vi "LEP_RV_StartInit.vi"(8 "error in (no error)":errorcluster, 9 "Application Name":string, 10 "Target Name":string, 11 "buildSpec ID":string) -> (0 "error out":errorcluster)   [LabVIEW 2011]
doc: "Download and execute built VxWorks downloadable module and attach the LabVIEW Embedded debuger."
uses:
  <vilib>/LabVIEW Targets/Embedded/ASWServer/MPU_ASWServer_GeneralIcons.ctl
  <vilib>/LabVIEW Targets/Embedded/ASWServer/MPU_ASWServer_GeneralCtrls.ctl
  <vilib>/LabVIEW Targets/Embedded/ASWServer/MPU_ASWServer_General_SetProgressBarTitle.vi
  <vilib>/LabVIEW Targets/Embedded/ASWServer/MPU_ASWServer_General_SetProgressBarValue.vi
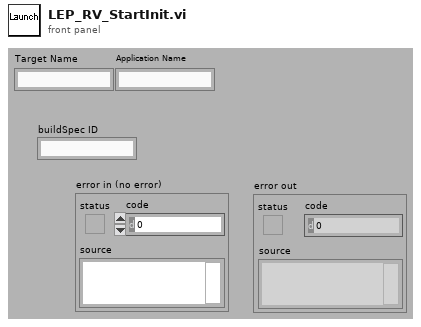
[diagram p1: front panel]
types:
  T1 = typedef "MPU_ASWServer_GeneralIcons.ctl" = enum16{"Complete", "Disconnected", "Error", "Initializing", "Ready", "Running", "Stopped", "Unknown", "No Change"}
  T2 = typedef "MPU_ASWServer_GeneralCtrls.ctl" = enum16{"Build Status", "Download Status", "Target Name", "Target Type", "Application Name"}
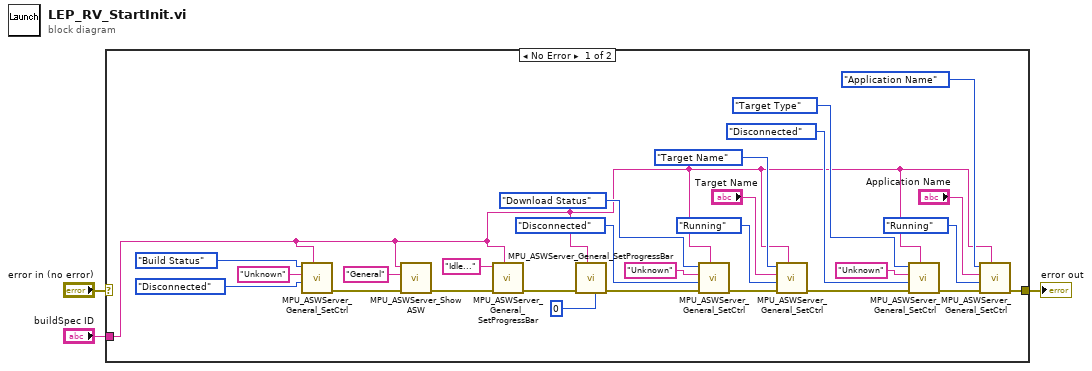
[diagram p0: block diagram]
diagram:
  n1 = case shown="No Error" "error in (no error)" {
    selector: "error in (no error)" -> [_ w31]
    tunnel: [w6 w31] -> w3
    tunnel: "buildSpec ID" -> [w8 _]
    frame No Error {
      n2 = call <vilib>:"MPU_ASWServer_General_SetCtrl.vi"("buildSpec ID"=w8, "icon"=MPU_ASWServer_GeneralIcons."Disconnected", "value"="Unknown", "control"=MPU_ASWServer_GeneralCtrls."Build Status") -> ("error out"=w5:errorcluster)  [unwired: 5 in, 2 out]
      n3 = call <vilib>:"MPU_ASWServer_Show ASW.vi"("error in (no error)"=w5, "tab name"="General", "buildSpec ID"=w8) -> ("error out"=w4:errorcluster)  [unwired: 7 in, 1 out]
      n4 = call-poly <vilib>:"MPU_ASWServer_General_SetProgressBar.vi"("buildSpec ID"=w8, "error in"=w4, "title"="Idle...") -> ("error out"=w30:errorcluster)  [unwired: 6 in, 2 out]
      n5 = call-poly <vilib>:"MPU_ASWServer_General_SetProgressBar.vi"("value"=u32 0, "buildSpec ID"=w8, "error in"=w30) -> ("error out"=w9:errorcluster)  [unwired: 6 in, 2 out]
      n6 = call <vilib>:"MPU_ASWServer_General_SetCtrl.vi"("buildSpec ID"=w8, "error in"=w9, "icon"=MPU_ASWServer_GeneralIcons."Disconnected", "value"="Unknown", "control"=MPU_ASWServer_GeneralCtrls."Download Status") -> ("error out"=w13:errorcluster)  [unwired: 4 in, 2 out]
      n7 = call <vilib>:"MPU_ASWServer_General_SetCtrl.vi"("buildSpec ID"=w8, "error in"=w13, "icon"=MPU_ASWServer_GeneralIcons."Running", "value"="Target Name", "control"=MPU_ASWServer_GeneralCtrls."Target Name") -> ("error out"=w15:errorcluster)  [unwired: 4 in, 2 out]
      n8 = call <vilib>:"MPU_ASWServer_General_SetCtrl.vi"("buildSpec ID"=w8, "error in"=w15, "icon"=MPU_ASWServer_GeneralIcons."Disconnected", "value"="Unknown", "control"=MPU_ASWServer_GeneralCtrls."Target Type") -> ("error out"=w11:errorcluster)  [unwired: 4 in, 2 out]
      n9 = call <vilib>:"MPU_ASWServer_General_SetCtrl.vi"("buildSpec ID"=w8, "error in"=w11, "icon"=MPU_ASWServer_GeneralIcons."Running", "value"="Application Name", "control"=MPU_ASWServer_GeneralCtrls."Application Name") -> ("error out"=w6:errorcluster)  [unwired: 4 in, 2 out]
    }
    frame Error {
    }
  }
  "error out" <- w3
